vi "plot_close.vi"(11 "Close?":bool) -> ()   [LabVIEW 2019]
panel:
  # "*******************************************************************\nBiogas Plant Control\n\nAuthor: Paul Zügel\nGCSC-Frankfurt am Main 2020\n\n*******************************************************************"
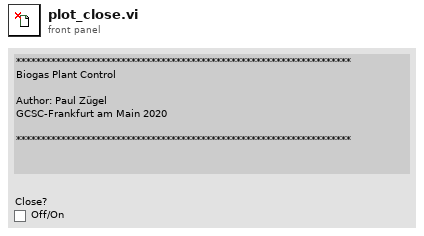
[diagram p1: front panel]
types:
  T1 = enum32{"Invalid", "Standard", "Closed", "Hidden", "Minimized", "Maximized"}
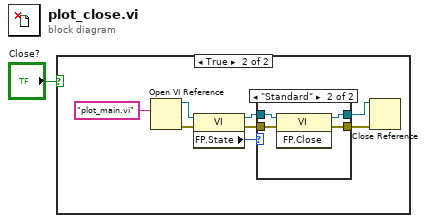
[diagram p0: block diagram]
diagram:
  n1 = case shown="True" "Close?" {
    frame False {
    }
    frame True {
      n2 = Open VI Reference(vi path="plot_main.vi") -> (vi reference=w8:refnum<vi>, error out=w9:errorcluster)  [unwired: 5 in]
      n3 = property class="VI"(reference=w8, error in=w9) -> (reference out=w6:refnum<vi>, error out=w7:errorcluster, "FP.State"=w5:T1)
      n4 = case shown="\"Standard\"" w5 {
        tunnel: w6 -> [w11 w15]
        tunnel: w7 -> [w10 w14]
        tunnel: [w11 w13] -> w2
        tunnel: [w10 w12] -> w3
        frame "Invalid", Default {
        }
        frame "Standard" {
          n5 = invoke class="VI" method="FP.Close"(reference=w15, error in=w14) -> (reference out=w13:refnum<vi>, error out=w12:errorcluster)  [unwired: 1 in, 1 out]
        }
      }
      n6 = Close Reference(reference=w2, error in (no error)=w3) -> ()  [unwired: 1 out]
    }
  }
